vi "Append Logger List.vi"(8 "error in (no error)":errorcluster, 10 "log":string[](array[string]), 11 "Logger Normal in":refnum<class "Logger Normal.lvclass">) -> (0 "error out":errorcluster, 3 "Logger Normal out":refnum<class "Logger Normal.lvclass">)   [LabVIEW 2020, in "Logger Normal.lvlib" / "Logger Normal.lvclass"]
uses:
  Logger Normal.lvclass
  Logger Normal Messages/Insert Log Msg/Insert Log Msg.lvclass
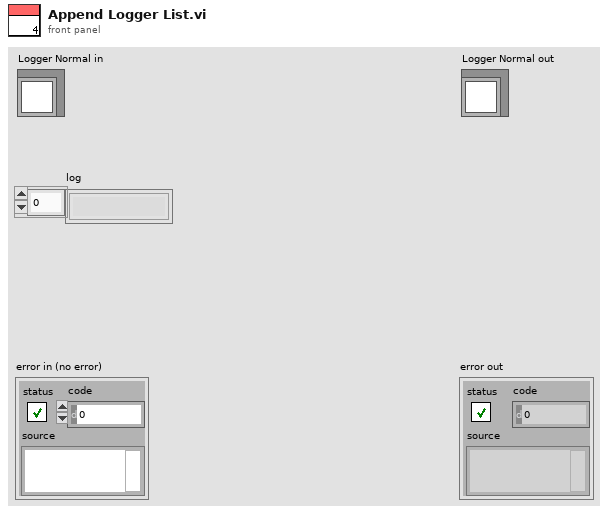
[diagram p1: front panel]
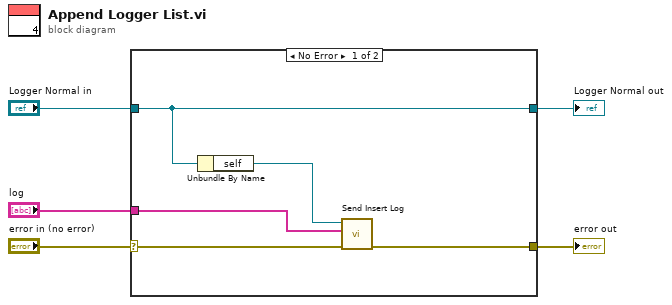
[diagram p0: block diagram]
diagram:
  n1 = case shown="No Error" "error in (no error)" {
    selector: "error in (no error)" -> [w9 w12]
    tunnel: [w6 w12] -> w4
    tunnel: [w10 w11] -> w2
    tunnel: "Logger Normal in" -> [w10 w11]
    tunnel: "log" -> [w7 _]
    frame No Error {
      n2 = Unbundle By Name(w10) -> ("self"=w8:refnum<class "Message Enqueuer.lvclass">)
      n3 = call "Send Insert Log.vi"("error in (no error)"=w9, "log"=w7, "Message Enqueuer"=w8) -> ("error out"=w6:errorcluster)  [unwired: 7 in, 1 out]
    }
    frame Error {
    }
  }
  "error out" <- w4
  "Logger Normal out" <- w2
